vi "New TCP Connection.vi"(8 "error in (no error)":errorcluster, 9 "remote port":u16, 10 "remote address":string, 11 "connection ID":refnum<k5>) -> (0 "error out":errorcluster, 3 "TCP Connection out":refnum<class "TCP Connection.lvclass">)   [LabVIEW 2019, in "TCP Connection.lvclass"]
doc: "<b>Description</b> Initialize a TCP Connection from a raw TCP connection refnum.\n\nBSD 3-Clause License\n\nCopyright (c) 2021, TauTerra, LLC\nAll rights reserved.\n\nRedistribution and use in source and binary forms, with or without\nmodification, are permitted provided that the following conditions are met:\n\n1. Redistributions of source code must retain the above copyright notice, this\n list of conditions and the following disclaimer.\n\n2. Redistributions in binary form must reproduce the above copyright notice,\n this list of conditions and the following disclaimer in the documentation\n and/or other materials provided with the distribution.\n\n3. Neither the name of the copyright holder nor the names of its\n contributors may be used to endorse or promote products derived from\n this software without specific prior written permission.\n\nTHIS SOFTWARE IS PROVIDED BY THE COPYRIGHT HOLDERS AND CONTRIBUTORS \"AS IS\"\nAND ANY EXPRESS OR IMPLIED WARRANTIES, INCLUDING, BUT NOT LIMITED TO, THE\nIMPLIED WARRANTIES OF MERCHANTABILITY AND FITNESS FOR A PARTICULAR PURPOSE ARE\nDISCLAIMED. IN NO EVENT SHALL THE COPYRIGHT HOLDER OR CONTRIBUTORS BE LIABLE\nFOR ANY DIRECT, INDIRECT, INCIDENTAL, SPECIAL, EXEMPLARY, OR CONSEQUENTIAL\nDAMAGES (INCLUDING, BUT NOT LIMITED TO, PROCUREMENT OF SUBSTITUTE GOODS OR\nSERVICES; LOSS OF USE, DATA, OR PROFITS; OR BUSINESS INTERRUPTION) HOWEVER\nCAUSED AND ON ANY THEORY OF LIABILITY, WHETHER IN CONTRACT, STRICT LIABILITY,\nOR TORT (INCLUDING NEGLIGENCE OR OTHERWISE) ARISING IN ANY WAY OUT OF THE USE\nOF THIS SOFTWARE, EVEN IF ADVISED OF THE POSSIBILITY OF SUCH DAMAGE."
uses:
  TCP Connection.lvclass
  TCP Connection.lvclass/TCP Connection.ctl
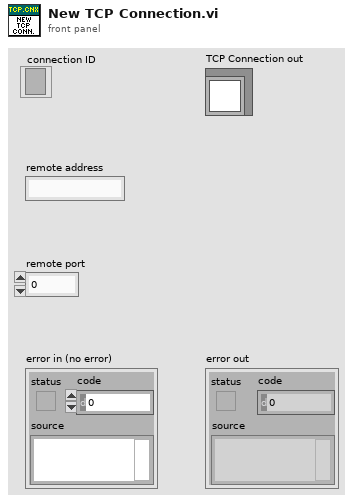
[diagram p1: front panel]
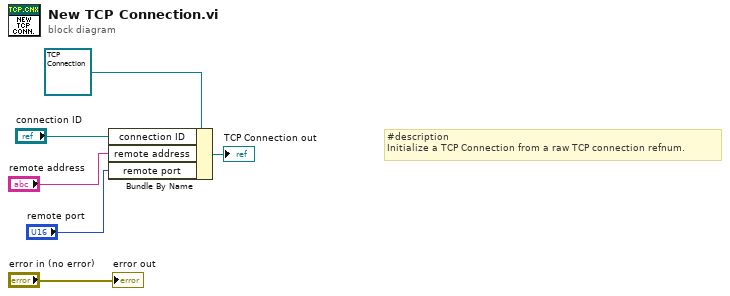
[diagram p0: block diagram]
diagram:
  # "#description\nInitialize a TCP Connection from a raw TCP connection refnum."
  n1 = Bundle By Name(cluster=refnum<class "TCP Connection.lvclass"> refnum ("TCP Connection out"), "connection ID"="connection ID", "remote address"="remote address", "remote port"="remote port") -> (→"TCP Connection out":refnum<class "TCP Connection.lvclass">)
  "error out" <- "error in (no error)"
